vi "test_BuildBinaries.vi"() -> (3 "Pass?":bool)   [LabVIEW 2019, in "Tests.General.lvlib"]
uses:
  Tests.General.lvlib
  <vilib>/AppBuilder/AB_API_Simple/Build (path).vi
  <vilib>/regexp/Match Regular Expression.xnode
  <vilib>/AppBuilder/AB_API_Simple/NI_App_Builder_API.lvlib
panel:
  out "error out":errorcluster
  out "Generated files":path[](array[path])
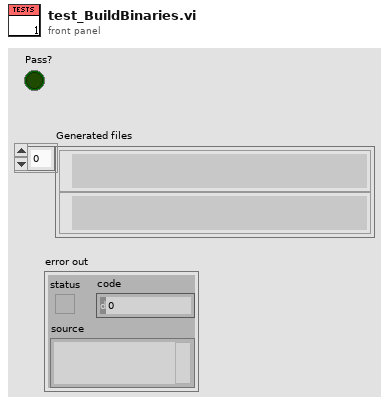
[diagram p1: front panel]
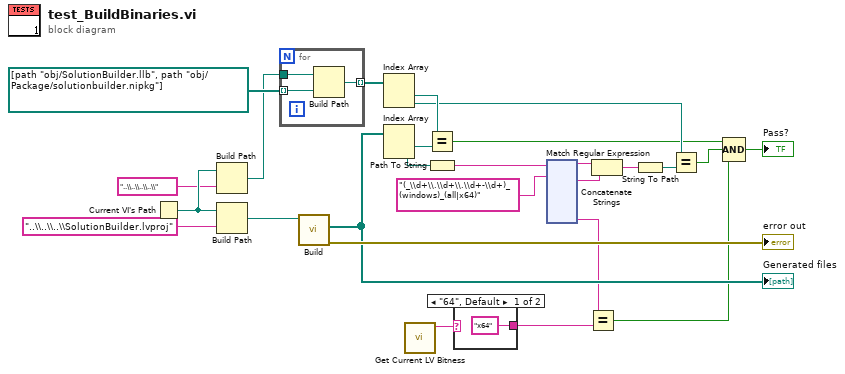
[diagram p0: block diagram]
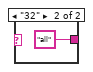
[diagram p2: hidden frame]
diagram:
  n1 = Current VI's Path() -> (path=w23:path)
  n2 = Build Path(base path=w23, name or relative path="..\\..\\..\\..\\") -> (appended path=w20:path)
  n3 = Build Path(base path=w23, name or relative path="..\\..\\..\\SolutionBuilder.lvproj") -> (appended path=w25:path)
  n4 = for {
    tunnel: path[] [path "obj/SolutionBuilder.llb", path "obj/Package/solutionbuilder.nipkg"] ("Generated files 2") -> [w28] mode=indexing
    tunnel: w20 -> [w29]
    tunnel: [w27] -> w19 mode=indexing
    n5 = Build Path(base path=w29, name or relative path=w28) -> (appended path=w27:path)
  }
  n6 = call-poly <vilib>:"Build.vi"("Path to project"=w25) -> ("error out"=→"error out":errorcluster, "Generated files"=w17:path[])  [unwired: 9 in]
  "Generated files" <- w17
  n7 = Index Array(array=w19) -> (element #1=w18:path, element #2=w8:path)  [unwired: 2 in]
  n8 = Index Array(array=w17) -> (element #1=w16:path, element #2=w15:path)  [unwired: 2 in]
  n9 = call <vilib>:"Get Current LV Bitness.vi"() -> ("bitness"=w4:string)  [unwired: 11 in]
  n10 = Equal?(x=w18, y=w16) -> (x = y?=w7:bool)
  n11 = Path To String(path=w15) -> (string=w13:string)
  n12 = case shown="\"64\", Default" w4 {
    tunnel: ["x64" ("name or relative path") "all" ("name or relative path")] -> w2
    frame "64", Default {
    }
    frame "32" {
    }
  }
  n13 = xnode "Match Regular Expression"("input string"=w13, "regular expression"="(_\\d+\\.\\d+\\.\\d+-\\d+)_(windows)_(all|x64)") -> ("before match"=w12:string, "after match"=w11:string, "submatch 3"=w3:string)  [unwired: 4 in, 5 out]
  n14 = Equal?(x=w3, y=w2) -> (x = y?=w1:bool)
  n15 = Concatenate Strings(w12, w11) -> (w10:string)
  n16 = String To Path(string=w10) -> (path=w9:path)
  n17 = Equal?(x=w8, y=w9) -> (x = y?=w6:bool)
  n18 = Compound Arithmetic op=AND(w7, w6, w1) -> (→"Pass?":bool)
